vi "RSZVB Set Coherent Signal Amplitude.vi"(7 "Amplitude (0.0 dB)":dbl format="%^.3e", 8 "error in (no error)":errorcluster {"code" format="%.0x"}, 9 "Port (1)":i32=1, 10 "Channel (1)":i32=1, 11 "VISA session":refnum<visa-resource-name>) -> (0 "error out":errorcluster {"code" format="%.0x"}, 3 "dup VISA session":refnum<visa-resource-name>)   [LabVIEW 2011]
doc: "This VI defines the amplitude for the coherent signal at port no. <Pt> relative to the amplitude of the reference signal (SOURce<Ch>:CMODe:RPORt). The amplitude replaces the port amplitude as long as the port signal is selected as a coherent signal (SOURce<Ch>:CMODe:PORT<Pt>[:STATe] ON). \n\nNote(s):\n\n(1) This VI is not available for R&S ZVB instrument.\n\nRemote-control command(s):\nSOURce<Ch>:CMODe:PORT<Pt>:AMPLitude"
uses:
  _utility/RSZVB Global Data.vi
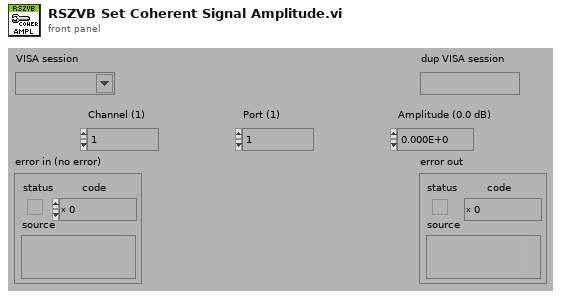
[diagram p1: front panel]
types:
  T1 = cluster{"Error Checking (T: On)":bool, "Installed Options":string[], "Data Valid?":bool, "Ports":i32, "Model":string[], "Option Checking (T: On)":bool}[]
  T2 = cluster{"Error Checking (T: On)":bool, "Installed Options":string[], "Data Valid?":bool, "Ports":i32, "Model":string[], "Option Checking (T: On)":bool}
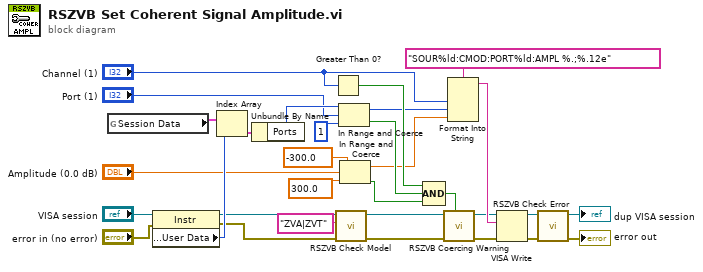
[diagram p0: block diagram]
diagram:
  n1 = global read "RSZVB Global Data.vi" "Session Data"() -> (w22:T1)
  n2 = property class="Instr"(reference="VISA session", error in="error in (no error)") -> (reference out=w1:refnum<visa-resource-name>, error out=w2:errorcluster, "General Settings:User Data"=w20:u32)
  n3 = Index Array(array=w22, index=w20) -> (element=w23:T2)
  n4 = Unbundle By Name(w23) -> ("Ports"=w19:i32)
  n5 = Greater Than 0?(x="Channel (1)") -> (x > 0?=w31:bool)
  n6 = call "RSZVB Check Model.vi"("error in (no error)"=w2, "Model"="ZVA|ZVT", "VISA session"=w1) -> ("error out"=w3:errorcluster, "dup VISA session"=w4:refnum<visa-resource-name>)  [unwired: 7 in]
  n7 = In Range and Coerce(upper limit=w19, x="Port (1)", lower limit=1) -> (coerced(x)=w18:i32, In Range?=w30:bool)
  n8 = In Range and Coerce(upper limit=-300.0 ("lower limit"), x="Amplitude (0.0 dB)", lower limit=300.0) -> (coerced(x)=w11:dbl, In Range?=w10:bool)
  n9 = Compound Arithmetic op=AND(w31, w30, w10) -> (w17:bool)
  n10 = call "RSZVB Coercing Warning.vi"("In Range?"=w17, "error in (no error)"=w3, "VISA session"=w4) -> ("error out"=w26:errorcluster, "dup VISA session"=w25:refnum<visa-resource-name>)  [unwired: 7 in]
  n11 = Format Into String(format string="SOUR%ld:CMOD:PORT%ld:AMPL %.;%.12e", "Channel (1)", w18, w11) -> (resulting string=w27:string)  [unwired: 2 in, 1 out]
  n12 = VISA Write(VISA resource name=w25, write buffer=w27, error in (no error)=w26) -> (VISA resource name out=w28:refnum<visa-resource-name>, error out=w29:errorcluster)  [unwired: 1 out]
  n13 = call "RSZVB Check Error.vi"("error in (no error)"=w29, "VISA session"=w28) -> ("error out"=→"error out":errorcluster, "dup VISA session"=→"dup VISA session":refnum<visa-resource-name>)  [unwired: 8 in]
